vi "Switch.vi"(8 "error in (no error)":errorcluster, 10 "Ref":string, 11 "Git Updater Module in":refnum<class "Git Updater Module.lvclass">) -> (0 "error out":errorcluster, 3 "Git Updater Module out":refnum<class "Git Updater Module.lvclass">)   [LabVIEW 2020, in "VolatusGUI.lvlib" / "Git Updater Module.lvclass"]
uses:
  Git Updater Module.lvclass
  <vilib>/Hampel Software Engineering/Git API/Git API/GIT-api.lvclass
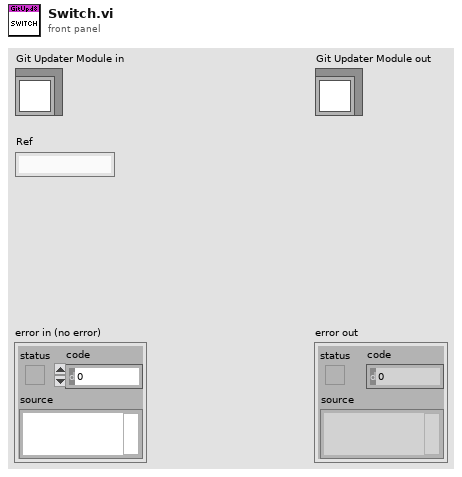
[diagram p1: front panel]
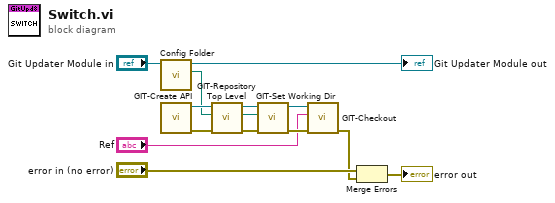
[diagram p0: block diagram]
diagram:
  n1 = call "Config Folder.vi"("Git Updater Module in"="Git Updater Module in") -> ("Config Folder"=w8:path, "Git Updater Module out"=→"Git Updater Module out":refnum<class "Git Updater Module.lvclass">)  [unwired: 8 in, 1 out]
  n2 = call <vilib>:"GIT-Create API.vi"() -> ("error out"=w12:errorcluster, "git-api out"=w13:refnum<class "GIT-api.lvclass">)  [unwired: 10 in]
  n3 = call <vilib>:"GIT-Repository Top Level.vi"("error in"=w12, "Current Path"=w8, "git-api in"=w13) -> ("error out"=w9:errorcluster, "Repo Top Level Path"=w10:path, "git-api out"=w11:refnum<class "GIT-api.lvclass">)  [unwired: 6 in]
  n4 = call <vilib>:"GIT-Set Working Dir.vi"("error in"=w9, "Working Directory"=w10, "git-api in"=w11) -> ("error out"=w5:errorcluster, "git-api out"=w4:refnum<class "GIT-api.lvclass">)  [unwired: 7 in]
  n5 = call <vilib>:"GIT-Checkout.vi"("error in"=w5, "branch name"="Ref", "git-api in"=w4) -> ("error out"=w1:errorcluster)  [unwired: 7 in, 1 out]
  n6 = Merge Errors("error in (no error)", w1) -> (→"error out":errorcluster)
